vi "Standard Event Status.vi"(6 "Set Parameter (0:Enable Reg)":T1(ring), 7 "Set/Check? (F:Set)":bool, 8 "error in (no error)":errorcluster, 9 "Check Parameter (0:Enable Reg)":T2(ring), 10 "Enable Value (0)":u16, 11 "VISA Resource Name":refnum<visa-resource-name>="GPIB0::9::INSTR") -> (0 "error out":errorcluster, 2 "Bits Set":bool[](array[boolean]), 3 "VISA Resource Name Out":refnum<visa-resource-name>)   [LabVIEW 2012, in "Agilent 34970.lvlib"]
doc: "This VI allows you to set or check the Standard Event registers."
uses:
  <instrlib>/Agilent 34970/Agilent 34970.lvlib
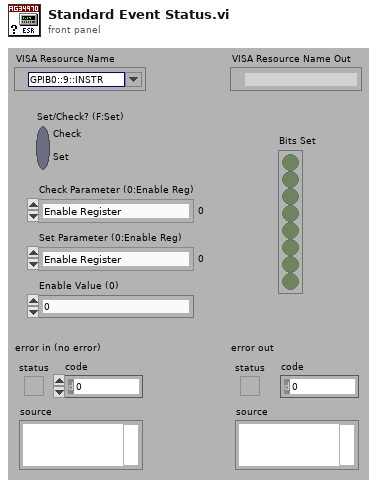
[diagram p1: front panel]
types:
  T1 = enum16{"Enable Register", "Operation Complete Bit"}
  T2 = enum16{"Enable Register", "Event Register", "Operation Complete Bit"}
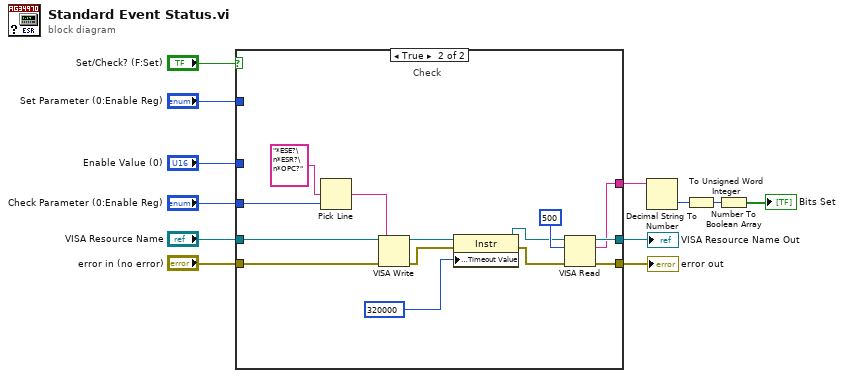
[diagram p0: block diagram]
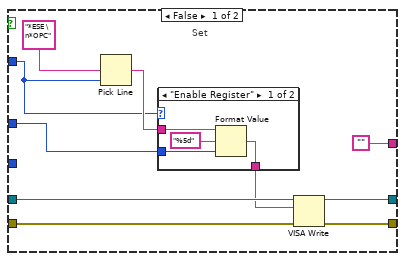
[diagram p2: hidden frame]
diagram:
  n1 = case shown="True" "Set/Check? (F:Set)" {
    tunnel: "Enable Value (0)" -> [w22 _]
    tunnel: "VISA Resource Name" -> [w21 w40]
    tunnel: "error in (no error)" -> [w20 w39]
    tunnel: [w19 w37] -> w3
    tunnel: [w18 w38] -> w2
    tunnel: "Check Parameter (0:Enable Reg)" -> [_ w34]
    tunnel: ["" w36] -> w9
    tunnel: "Set Parameter (0:Enable Reg)" -> [w14 _]
    frame False {
      # "Set"
      n2 = Pick Line(multi-line string="*ESE \n*OPC", line index=w14) -> (output string=w15:string)  [unwired: 1 in]
      n3 = case shown="\"Enable Register\"" w14 {
        tunnel: [w26 w27] -> w13
        tunnel: w15 -> [w25 w27]
        tunnel: w22 -> [w23 _]
        frame "Enable Register" {
          n4 = Format Value(string ("")=w25, format string="%5d", value (0)=w23) -> (output string=w26:string)
        }
        frame "Operation Complete Bit" {
        }
      }
      n5 = VISA Write(VISA resource name=w21, write buffer=w13, error in (no error)=w20) -> (VISA resource name out=w19:refnum<visa-resource-name>, error out=w18:errorcluster)  [unwired: 1 out]
    }
    frame True {
      # "Check"
      n6 = Pick Line(multi-line string="*ESE?\n*ESR?\n*OPC?", line index=w34) -> (output string=w35:string)  [unwired: 1 in]
      n7 = VISA Write(VISA resource name=w40, write buffer=w35, error in (no error)=w39) -> (VISA resource name out=w31:refnum<visa-resource-name>, error out=w30:errorcluster)  [unwired: 1 out]
      n8 = property class="Instr"(reference=w31, error in=w30, "General Settings:Timeout Value"=u32 320000 ("Tmo Value")) -> (reference out=w28:refnum<visa-resource-name>, error out=w29:errorcluster)
      n9 = VISA Read(VISA resource name=w28, byte count=u32 500 ("byte count (0)"), error in (no error)=w29) -> (VISA resource name out=w37:refnum<visa-resource-name>, read buffer=w36:string, error out=w38:errorcluster)  [unwired: 1 out]
    }
  }
  "error out" <- w2
  "VISA Resource Name Out" <- w3
  n10 = Decimal String To Number(string=w9) -> (number=w8:i32)  [unwired: 2 in, 1 out]
  n11 = To Unsigned Word Integer(number=w8) -> (unsigned 16bit integer=w7:u16)
  n12 = Number To Boolean Array(number=w7) -> (Boolean array=→"Bits Set":bool[])
